vi "Grab.vi"(8 "error in (no error)":errorcluster, 10 "Image":T1, 11 "Imaq Camera in":refnum<class "Imaq Camera.lvclass">) -> (0 "error out":errorcluster, 2 "Image out":T1, 3 "Imaq Camera out":refnum<class "Imaq Camera.lvclass">)   [LabVIEW 2022 SP3, in "Imaq Camera.lvclass"]
uses:
  Imaq Camera.lvclass
  <vilib>/vision/Image Controls.llb/IMAQ Image.ctl
  <vilib>/vision/driver/IMAQdx.llb/IMAQdx Buffer Number Mode.ctl
  Imaq Camera.lvclass/Imaq Camera.ctl
  <vilib>/vision/driver/NI_Vision_Acquisition_Software.lvlib
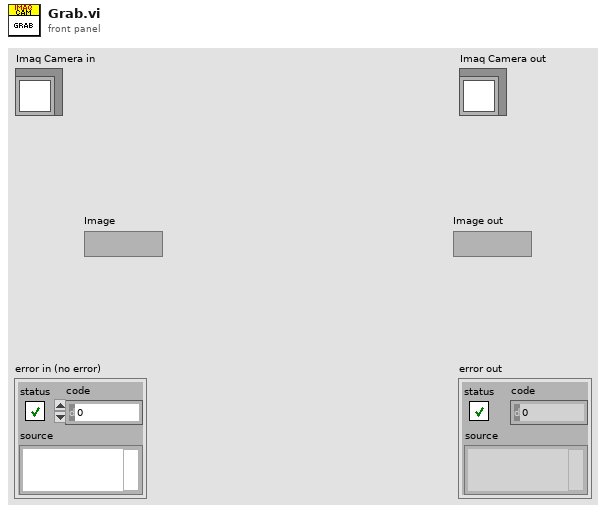
[diagram p1: front panel]
types:
  T1 = typedef "IMAQ Image.ctl" = refnum<image>
  T2 = typedef "NI_Vision_Acquisition_Software.lvlib/IMAQdx Buffer Number Mode.ctl" = enum32{"Next", "Last", "Buffer Number", "Every", "Last New"}
  T3 = typedef "IMAQdx.ctl" = refnum<k21>
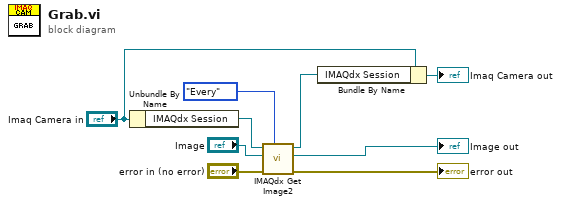
[diagram p0: block diagram]
diagram:
  n1 = Unbundle By Name("Imaq Camera in") -> ("IMAQdx Session"=w6:T3)
  n2 = call <vilib>:"IMAQdx Get Image2.vi"("Buffer Number Mode (Next)"=IMAQdx_Buffer_Number_Mode."Every" ("Buffer Number Mode"), "error in"="error in (no error)", "Image In"="Image", "Session In"=w6) -> ("error out"=→"error out":errorcluster, "Image Out"=→"Image out":T1, "Session Out"=w3:T3)  [unwired: 4 in, 1 out]
  n3 = Bundle By Name(cluster="Imaq Camera in", "IMAQdx Session"=w3) -> (→"Imaq Camera out":refnum<class "Imaq Camera.lvclass">)
